vi "CLOSE.vi"(11 "Pump_1AI_1DO_2DI in":refnum<class "ValveModbus.lvclass">) -> (3 "Pump_1AI_1DO_2DI out":refnum<class "ValveModbus.lvclass">)   [LabVIEW 2019, in "ValveModbus.lvclass"]
uses:
  ValveModbus.lvclass
  ValveModbus.lvclass/ValveModbus.ctl
  TypeDef/StateValveModbus.ctl
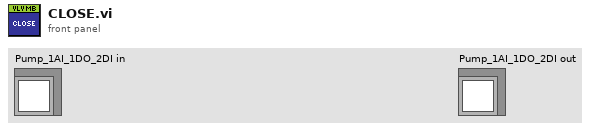
[diagram p1: front panel]
types:
  T1 = typedef "StateValveModbus.ctl" = enum16{"IDLE", "OPEN", "CLOSE", "OPENING", "CLOSING", "STOP"}
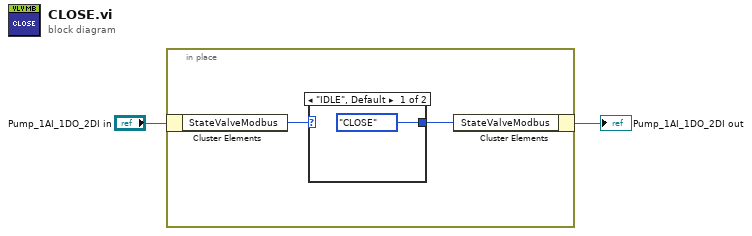
[diagram p0: block diagram]
diagram:
  n1 = in-place {
    n2 = in-place-cluster #1("Pump_1AI_1DO_2DI in") -> ("StateValveModbus"=w3:T1)
    n3 = case shown="\"IDLE\", Default" w3 {
      selector: w3 -> [_ w6]
      tunnel: [StateValveModbus."CLOSE" ("StateValveModbus") w6] -> w4
      frame "IDLE", Default {
      }
      frame "CLOSE", "CLOSING" {
      }
    }
    n4 = in-place-cluster #1("StateValveModbus"=w4) -> (→"Pump_1AI_1DO_2DI out":refnum<class "ValveModbus.lvclass">)
  }
